vi "Target3.vi"   [LabVIEW 2025]
uses:
  <vilib>/eio/utilities/niEioResolveVilibRelativePath.vi
  <vilib>/rvi/interface/RandomDataEmulation/niFpgaRandomDataHandleErrors.vi
  <vilib>/rvi/Memory/Memory_Emulation/nirvimemoryFastEmulation.vi
  <vilib>/rvi/Memory/Memory_Emulation/nirvimemoryEmulation.vi
  <vilib>/rvi/Emulation/niFpgaEmulationIsFPGAContextNoSignature.vi
  <vilib>/rvi/DataTransferAndStorage/Container/Common/niFpgaContainerGetUniqueNameForEmu.vi
  <vilib>/rvi/Emulation/niFpgaProcessEmulError.vi
  <vilib>/rvi/Emulation/niFpgaSctlEmulationGetInTimedLoop.vi
  <vilib>/rvi/errors/nirviReportUnexpectedCaseInternalError (U32).vi
  <vilib>/rvi/DataTransferAndStorage/Container/XNode/niFpgaContainer.xnode
  <vilib>/rvi/interface/RandomDataEmulation/nirviRandomDataFpgaReadWriteTemplate.vi
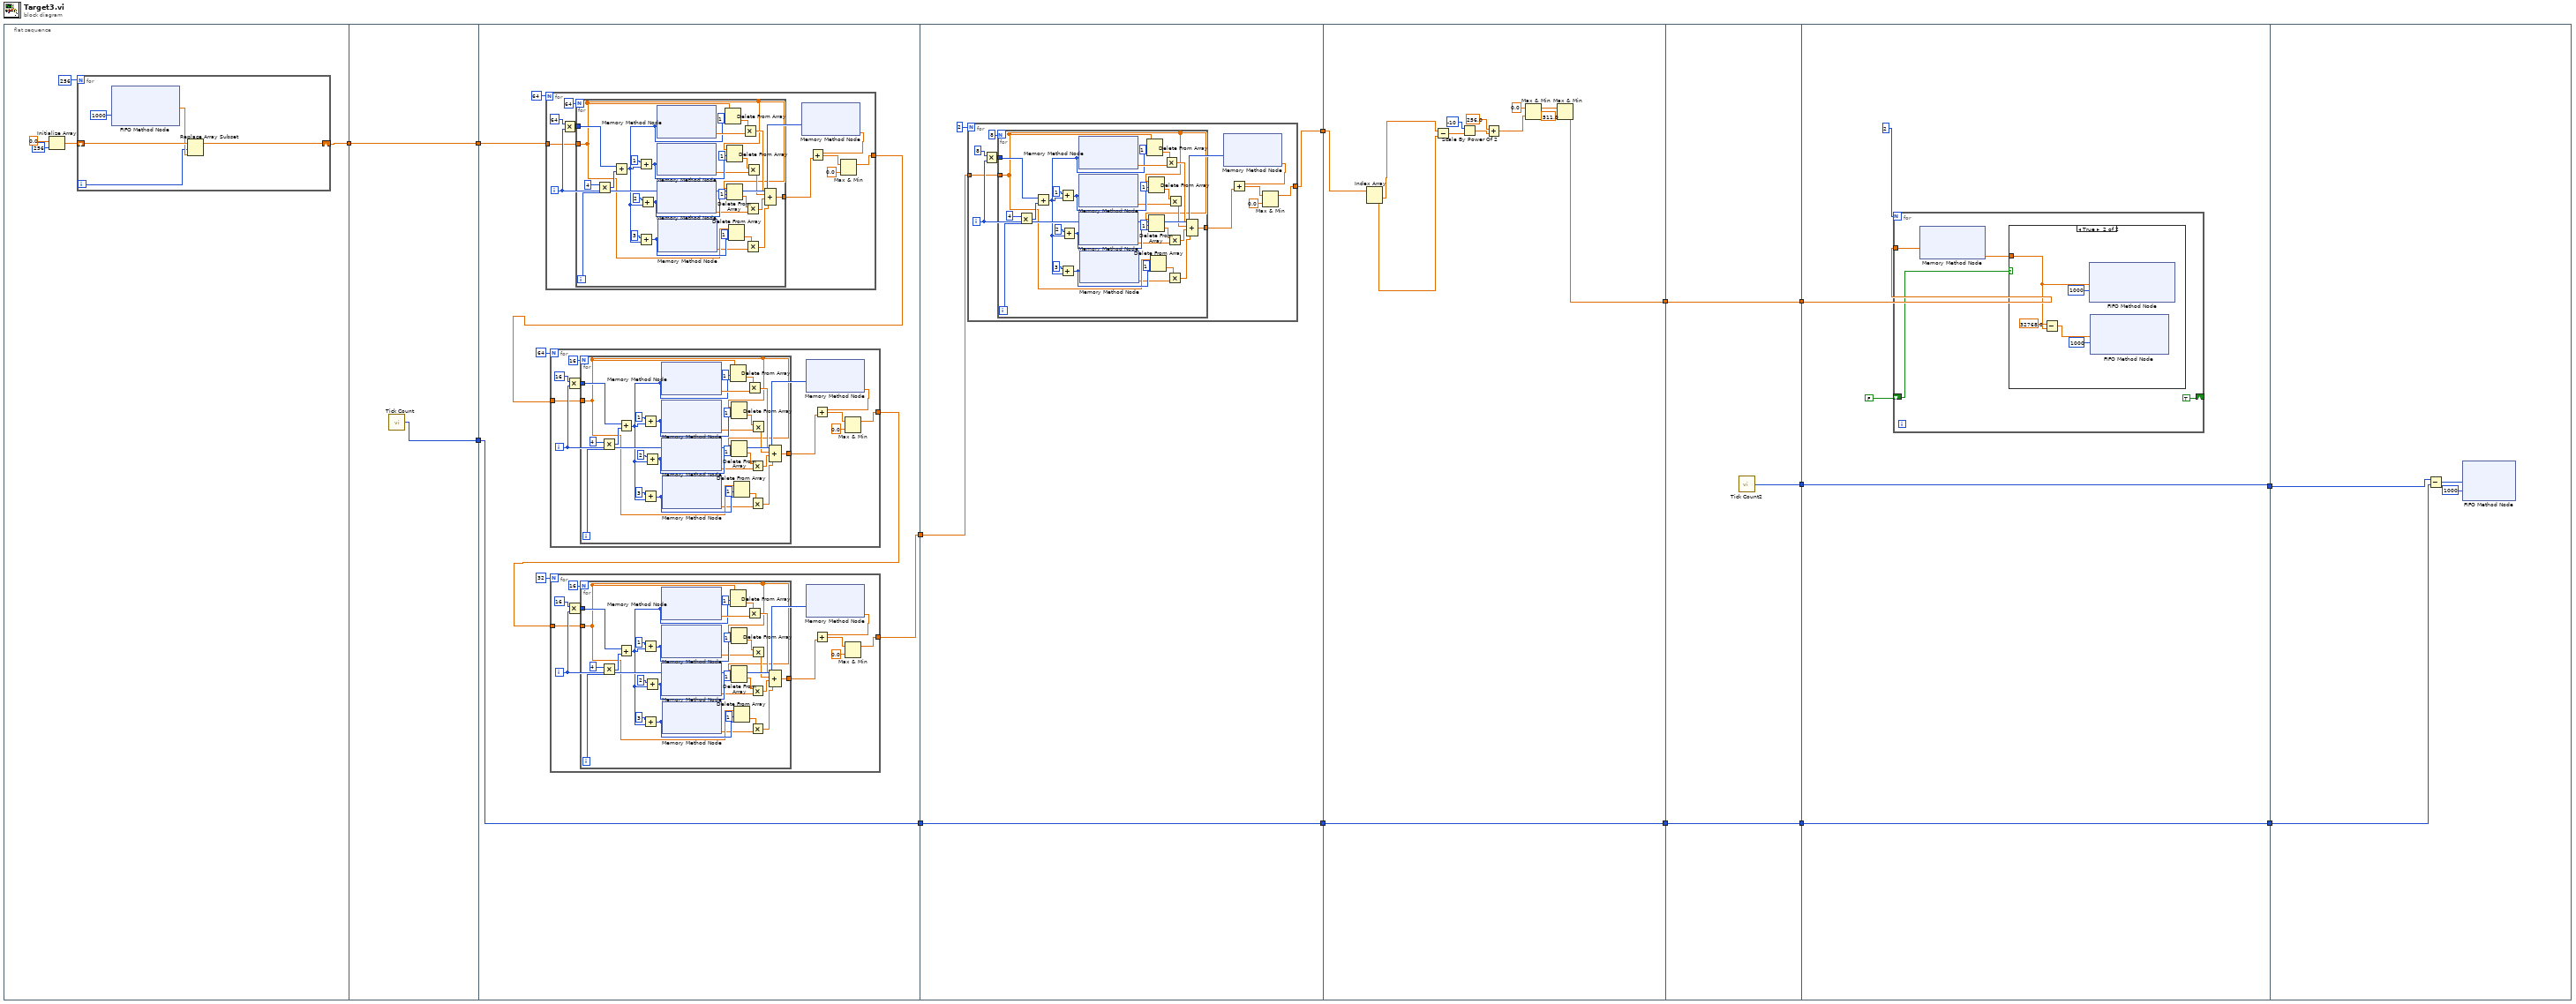
[diagram p0: block diagram]
diagram:
  n1 = flat-sequence {
    tunnel: [w18] -> w14
    tunnel: w14 -> [w26]
    tunnel: [w26] -> w13
    tunnel: [w25] -> w12
    tunnel: w13 -> [w33]
    tunnel: [w28] -> w11
    tunnel: w12 -> [w27]
    tunnel: [w27] -> w1
    tunnel: w11 -> [w153]
    tunnel: [w152] -> w10
    tunnel: [w155] -> w2
    tunnel: w1 -> [w155]
    tunnel: w10 -> [w197]
    tunnel: [w196] -> w9
    tunnel: [w195] -> w3
    tunnel: w2 -> [w195]
    tunnel: w9 -> [w210]
    tunnel: [w210] -> w8
    tunnel: [w209] -> w7
    tunnel: [w208] -> w4
    tunnel: w3 -> [w208]
    tunnel: w8 -> [w214]
    tunnel: [w212] -> w6
    tunnel: w7 -> [w212]
    tunnel: [w211] -> w5
    tunnel: w4 -> [w211]
    tunnel: w6 -> [w228]
    tunnel: w5 -> [w225]
    frame #0 {
      n2 = Initialize Array(sgl 0.0 ("element"), 256 ("dimension size")) -> (w15:sgl[])
      n3 = for {
        N: 256 -> [_]
        shift-right: [w21] -> w18
        shift-left: w15 -> [w23]
        i -> [w20]
        n4 = xnode ("FIFO Method Node")("Timeout"=1000) -> ("Element"=w22:sgl)  [unwired: 1 in, 2 out]
        n5 = Replace Array Subset(array=w23, new element=w22, index=w20) -> (w21:sgl[])
      }
    }
    frame #1 {
      n6 = call "Tick Count"() -> ("Tick Count(uSec)"=w25:u32)
    }
    frame #2 {
      n7 = for {
        N: 64 -> [_]
        tunnel: w33 -> [w114]
        tunnel: [w115] -> w31
        i -> [w119]
        n8 = Multiply(x=64, y=w119) -> (x*y=w118:i32)
        n9 = for {
          N: 64 -> [_]
          tunnel: w118 -> [w151]
          tunnel: w114 -> [w127]
          tunnel: [w123] -> w113
          i -> [w150]
          n10 = Multiply(x=4, y=w150) -> (x*y=w148:i32)
          n11 = Add(x=w151, y=w148) -> (x+y=w142:i32)
          n12 = Add(x=1, y=w142) -> (x+y=w133:i32)
          n13 = Add(x=3, y=w142) -> (x+y=w131:i32)
          n14 = Add(x=2, y=w142) -> (x+y=w132:i32)
          n15 = xnode ("Memory Method Node")("Address"=w142) -> ("Data"=w143:sgl)  [unwired: 1 in, 1 out]
          n16 = xnode ("Memory Method Node")("Address"=w133) -> ("Data"=w128:sgl)  [unwired: 1 in, 1 out]
          n17 = xnode ("Memory Method Node")("Address"=w132) -> ("Data"=w124:sgl)  [unwired: 1 in, 1 out]
          n18 = xnode ("Memory Method Node")("Address"=w131) -> ("Data"=w125:sgl)  [unwired: 1 in, 1 out]
          n19 = Delete From Array(array=w127, length=1, index=w142) -> (deleted portion=w144:sgl[])  [unwired: 1 out]
          n20 = Delete From Array(array=w127, length=1, index=w133) -> (deleted portion=w129:sgl[])  [unwired: 1 out]
          n21 = Delete From Array(array=w127, length=1, index=w132) -> (deleted portion=w130:sgl[])  [unwired: 1 out]
          n22 = Delete From Array(array=w127, length=1, index=w131) -> (deleted portion=w126:sgl[])  [unwired: 1 out]
          n23 = Multiply(x=w144, y=w143) -> (x*y=w137:sgl[])
          n24 = Multiply(x=w130, y=w124) -> (x*y=w135:sgl[])
          n25 = Multiply(x=w126, y=w125) -> (x*y=w134:sgl[])
          n26 = Multiply(x=w129, y=w128) -> (x*y=w136:sgl[])
          n27 = Compound Arithmetic op=ADD(w137, w136, w135, w134) -> (w123:sgl[])
        }
        n28 = xnode ("Memory Method Node")("Address"=w119) -> ("Data"=w121:sgl)  [unwired: 1 in, 1 out]
        n29 = Add(x=w121, y=w113) -> (x+y=w117:sgl[])
        n30 = Max & Min(x=w117, y=sgl 0.0) -> (max(x,y)=w115:sgl[])  [unwired: 1 out]
      }
      n31 = for {
        N: 64 -> [_]
        tunnel: w31 -> [w75]
        tunnel: [w76] -> w29
        i -> [w80]
        n32 = Multiply(x=16, y=w80) -> (x*y=w79:i32)
        n33 = for {
          N: 16 -> [_]
          tunnel: w79 -> [w112]
          tunnel: w75 -> [w88]
          tunnel: [w84] -> w74
          i -> [w111]
          n34 = Multiply(x=4, y=w111) -> (x*y=w109:i32)
          n35 = Add(x=w112, y=w109) -> (x+y=w103:i32)
          n36 = Add(x=1, y=w103) -> (x+y=w94:i32)
          n37 = Add(x=3, y=w103) -> (x+y=w92:i32)
          n38 = Add(x=2, y=w103) -> (x+y=w93:i32)
          n39 = xnode ("Memory Method Node")("Address"=w103) -> ("Data"=w104:sgl)  [unwired: 1 in, 1 out]
          n40 = xnode ("Memory Method Node")("Address"=w94) -> ("Data"=w89:sgl)  [unwired: 1 in, 1 out]
          n41 = xnode ("Memory Method Node")("Address"=w93) -> ("Data"=w85:sgl)  [unwired: 1 in, 1 out]
          n42 = xnode ("Memory Method Node")("Address"=w92) -> ("Data"=w86:sgl)  [unwired: 1 in, 1 out]
          n43 = Delete From Array(array=w88, length=1, index=w103) -> (deleted portion=w105:sgl[])  [unwired: 1 out]
          n44 = Delete From Array(array=w88, length=1, index=w94) -> (deleted portion=w90:sgl[])  [unwired: 1 out]
          n45 = Delete From Array(array=w88, length=1, index=w93) -> (deleted portion=w91:sgl[])  [unwired: 1 out]
          n46 = Delete From Array(array=w88, length=1, index=w92) -> (deleted portion=w87:sgl[])  [unwired: 1 out]
          n47 = Multiply(x=w105, y=w104) -> (x*y=w98:sgl[])
          n48 = Multiply(x=w91, y=w85) -> (x*y=w96:sgl[])
          n49 = Multiply(x=w87, y=w86) -> (x*y=w95:sgl[])
          n50 = Multiply(x=w90, y=w89) -> (x*y=w97:sgl[])
          n51 = Compound Arithmetic op=ADD(w98, w97, w96, w95) -> (w84:sgl[])
        }
        n52 = xnode ("Memory Method Node")("Address"=w80) -> ("Data"=w82:sgl)  [unwired: 1 in, 1 out]
        n53 = Add(x=w82, y=w74) -> (x+y=w78:sgl[])
        n54 = Max & Min(x=w78, y=sgl 0.0) -> (max(x,y)=w76:sgl[])  [unwired: 1 out]
      }
      n55 = for {
        N: 32 -> [_]
        tunnel: w29 -> [w36]
        tunnel: [w37] -> w28
        i -> [w41]
        n56 = Multiply(x=16, y=w41) -> (x*y=w40:i32)
        n57 = for {
          N: 16 -> [_]
          tunnel: w40 -> [w73]
          tunnel: w36 -> [w49]
          tunnel: [w45] -> w35
          i -> [w72]
          n58 = Multiply(x=4, y=w72) -> (x*y=w70:i32)
          n59 = Add(x=w73, y=w70) -> (x+y=w64:i32)
          n60 = Add(x=1, y=w64) -> (x+y=w55:i32)
          n61 = Add(x=3, y=w64) -> (x+y=w53:i32)
          n62 = Add(x=2, y=w64) -> (x+y=w54:i32)
          n63 = xnode ("Memory Method Node")("Address"=w64) -> ("Data"=w65:sgl)  [unwired: 1 in, 1 out]
          n64 = xnode ("Memory Method Node")("Address"=w55) -> ("Data"=w50:sgl)  [unwired: 1 in, 1 out]
          n65 = xnode ("Memory Method Node")("Address"=w54) -> ("Data"=w46:sgl)  [unwired: 1 in, 1 out]
          n66 = xnode ("Memory Method Node")("Address"=w53) -> ("Data"=w47:sgl)  [unwired: 1 in, 1 out]
          n67 = Delete From Array(array=w49, length=1, index=w64) -> (deleted portion=w66:sgl[])  [unwired: 1 out]
          n68 = Delete From Array(array=w49, length=1, index=w55) -> (deleted portion=w51:sgl[])  [unwired: 1 out]
          n69 = Delete From Array(array=w49, length=1, index=w54) -> (deleted portion=w52:sgl[])  [unwired: 1 out]
          n70 = Delete From Array(array=w49, length=1, index=w53) -> (deleted portion=w48:sgl[])  [unwired: 1 out]
          n71 = Multiply(x=w66, y=w65) -> (x*y=w59:sgl[])
          n72 = Multiply(x=w52, y=w46) -> (x*y=w57:sgl[])
          n73 = Multiply(x=w48, y=w47) -> (x*y=w56:sgl[])
          n74 = Multiply(x=w51, y=w50) -> (x*y=w58:sgl[])
          n75 = Compound Arithmetic op=ADD(w59, w58, w57, w56) -> (w45:sgl[])
        }
        n76 = xnode ("Memory Method Node")("Address"=w41) -> ("Data"=w43:sgl)  [unwired: 1 in, 1 out]
        n77 = Add(x=w43, y=w35) -> (x+y=w39:sgl[])
        n78 = Max & Min(x=w39, y=sgl 0.0) -> (max(x,y)=w37:sgl[])  [unwired: 1 out]
      }
    }
    frame #3 {
      n79 = for {
        N: 2 -> [_]
        tunnel: w153 -> [w157]
        tunnel: [w158] -> w152
        i -> [w162]
        n80 = Multiply(x=8, y=w162) -> (x*y=w161:i32)
        n81 = for {
          N: 8 -> [_]
          tunnel: w161 -> [w194]
          tunnel: w157 -> [w170]
          tunnel: [w166] -> w156
          i -> [w193]
          n82 = Multiply(x=4, y=w193) -> (x*y=w191:i32)
          n83 = Add(x=w194, y=w191) -> (x+y=w185:i32)
          n84 = Add(x=1, y=w185) -> (x+y=w176:i32)
          n85 = Add(x=3, y=w185) -> (x+y=w174:i32)
          n86 = Add(x=2, y=w185) -> (x+y=w175:i32)
          n87 = xnode ("Memory Method Node")("Address"=w185) -> ("Data"=w186:sgl)  [unwired: 1 in, 1 out]
          n88 = xnode ("Memory Method Node")("Address"=w176) -> ("Data"=w171:sgl)  [unwired: 1 in, 1 out]
          n89 = xnode ("Memory Method Node")("Address"=w175) -> ("Data"=w167:sgl)  [unwired: 1 in, 1 out]
          n90 = xnode ("Memory Method Node")("Address"=w174) -> ("Data"=w168:sgl)  [unwired: 1 in, 1 out]
          n91 = Delete From Array(array=w170, length=1, index=w185) -> (deleted portion=w187:sgl[])  [unwired: 1 out]
          n92 = Delete From Array(array=w170, length=1, index=w176) -> (deleted portion=w172:sgl[])  [unwired: 1 out]
          n93 = Delete From Array(array=w170, length=1, index=w175) -> (deleted portion=w173:sgl[])  [unwired: 1 out]
          n94 = Delete From Array(array=w170, length=1, index=w174) -> (deleted portion=w169:sgl[])  [unwired: 1 out]
          n95 = Multiply(x=w187, y=w186) -> (x*y=w180:sgl[])
          n96 = Multiply(x=w173, y=w167) -> (x*y=w178:sgl[])
          n97 = Multiply(x=w169, y=w168) -> (x*y=w177:sgl[])
          n98 = Multiply(x=w172, y=w171) -> (x*y=w179:sgl[])
          n99 = Compound Arithmetic op=ADD(w180, w179, w178, w177) -> (w166:sgl[])
        }
        n100 = xnode ("Memory Method Node")("Address"=w162) -> ("Data"=w164:sgl)  [unwired: 1 in, 1 out]
        n101 = Add(x=w164, y=w156) -> (x+y=w160:sgl[])
        n102 = Max & Min(x=w160, y=sgl 0.0) -> (max(x,y)=w158:sgl[])  [unwired: 1 out]
      }
    }
    frame #4 {
      n103 = Index Array(array=w197) -> (element #1=w202:sgl, element #2=w203:sgl)  [unwired: 2 in]
      n104 = Subtract(x=w202, y=w203) -> (x-y=w204:sgl)
      n105 = Scale By Power Of 2(n=i16 -10, x=w204) -> (x*2^n=w205:sgl)
      n106 = Add(x=sgl 256.0, y=w205) -> (x+y=w206:sgl)
      n107 = Max & Min(x=sgl 0.0, y=w206) -> (max(x,y)=w207:sgl)  [unwired: 1 out]
      n108 = Max & Min(x=w207, y=sgl 511.0) -> (min(x,y)=w196:sgl)  [unwired: 1 out]
    }
    frame #5 {
      n109 = call "Tick Count2"() -> ("Tick Count(uSec)"=w209:u32)
    }
    frame #6 {
      n110 = for {
        N: 2 -> [_]
        tunnel: w214 -> [w219]
        shift-right: [TRUE] -> _
        shift-left: FALSE -> [w218]
        n111 = xnode ("Memory Method Node")("Address"=w219) -> ("Data"=w216:sgl)  [unwired: 1 in, 1 out]
        n112 = case shown="True" w218 {
          tunnel: w216 -> [_ w220]
          frame False {
          }
          frame True {
            n113 = Subtract(x=sgl 32768.0, y=w220) -> (x-y=w224:sgl)
            n114 = xnode ("FIFO Method Node")("Element"=w220, "Timeout"=1000) -> ()  [unwired: 1 in, 2 out]
            n115 = xnode ("FIFO Method Node")("Element"=w224, "Timeout"=1000) -> ()  [unwired: 1 in, 2 out]
          }
        }
      }
    }
    frame #7 {
      n116 = Subtract(x=w228, y=w225) -> (x-y=w227:u32)
      n117 = xnode ("FIFO Method Node")("Element"=w227, "Timeout"=1000) -> ()  [unwired: 1 in, 2 out]
    }
  }
